vi "Buffer Test.vi"() -> ()   [LabVIEW 2011]
uses:
  <vilib>/Instr/_visa.llb/VISA Configure Serial Port (Instr).vi
  <userlib>/Bloomy Controls/Timing/BCI_Timing.lvlib
panel:
  out "return count":u32
  out "read buffer":string
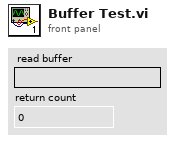
[diagram p1: front panel]
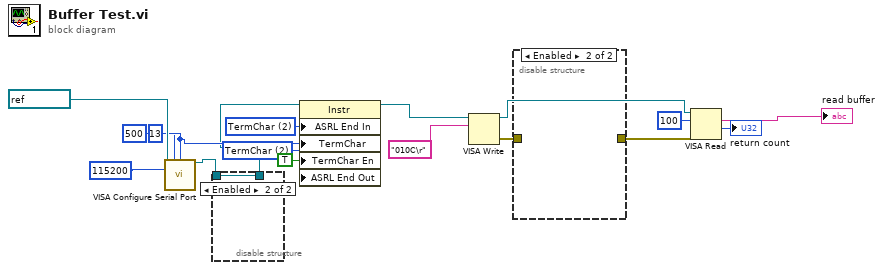
[diagram p0: block diagram]
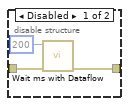
[diagram p2: hidden frame]
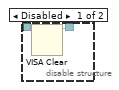
[diagram p3: hidden frame]
diagram:
  w1 = u16 2 items=["None", "Last Bit", "TermChar", "Break"] ("Serial Settings:End Mode for Writes")
  w16 = u16 2 items=["None", "Last Bit", "TermChar"] ("Serial Settings:End Mode for Reads")
  w6 = u8 13 ("termination char\n(0xA = '\\n' = LF)")
  n1 = call-poly "VISA Configure Serial Port"("VISA resource name"=refnum<visa-resource-name> "COM3", "timeout (10sec)"=u32 500, "termination char\n(0xA = '\\n' = LF)"=w6, "baud rate (9600)"=u32 115200) -> ("VISA resource name out"=w4:refnum<visa-resource-name>)  [unwired: 10 in, 1 out]
  n2 = disable-structure shown="Enabled" {
    disable-tunnel: w4 -> [w19 w20]
    disable-tunnel: [w18 w20] -> w3
    frame Disabled {
      n3 = VISA Clear(VISA resource name=w19) -> (VISA resource name out=w18:refnum<visa-resource-name>)  [unwired: 1 in, 1 out]
    }
    frame Enabled {
    }
  }
  n4 = property class="Instr"(reference=w3, "ASRL End In"=w16, "TermChar"=w6, "TermChar En"=TRUE ("Message Based Settings:Termination Character Enable"), "ASRL End Out"=w1) -> (reference out=w15:refnum<visa-resource-name>)  [unwired: 1 in, 1 out]
  n5 = VISA Write(VISA resource name=w15, write buffer="010C\r") -> (VISA resource name out=w11:refnum<visa-resource-name>, error out=w13:errorcluster)  [unwired: 1 in, 1 out]
  n6 = disable-structure shown="Enabled" {
    disable-tunnel: w13 -> [w23 _]
    disable-tunnel: [w21 _] -> w12
    frame Disabled {
      n7 = call <userlib>:"Wait ms with Dataflow.vi"("error in (no error)"=w23, "milliseconds to wait"=u32 200) -> ("error out"=w21:errorcluster)  [unwired: 8 in, 1 out]
    }
    frame Enabled {
    }
  }
  n8 = VISA Read(VISA resource name=w11, byte count=u32 100, error in (no error)=w12) -> (read buffer=→"read buffer":string, return count=→"return count":u32)  [unwired: 2 out]
